vi "Curtin1_ReadWriteFRFGraphData.vi"(8 "Type":T3 items=["FRF", "rad phase unwrapped", "deg phase unwrapped", "rad phase wrapped", "deg phase wrapped", "White Plots", "MJ Map", "Real and Imaginary"], 9 "FRF":refnum<vi>, 11 "Task":enum16{"Read", "Save"}(ring)) -> (0 "y log?":bool, 1 "x log?":bool, 2 "dB":dbl)   [LabVIEW 2022 SP3]
uses:
  GraphType.ctl
  <vilib>/Utility/miscctls.llb/LVRangeTypeDef.ctl
  Mic/Mic_Global.vi
panel:
  out "Graph settings":T2
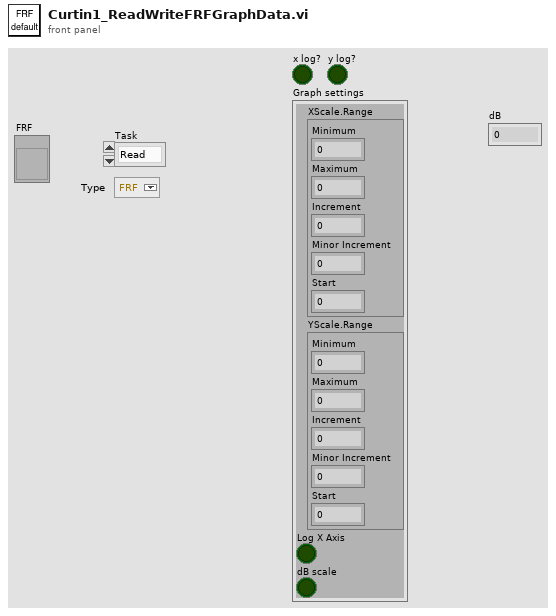
[diagram p1: front panel]
types:
  T1 = typedef "LVRangeTypeDef.ctl" = cluster{"Minimum":dbl, "Maximum":dbl, "Increment":dbl, "Minor Increment":dbl, "Start":dbl}
  T2 = cluster{"XScale.Range":T1, "YScale.Range":T1, "Log X Axis":bool, "dB scale":bool}
  T3 = typedef "GraphType.ctl" = u16
  T4 = cluster{"Alerts":bool, "Log X Axis":bool, "dB scale":bool, "Averaging":bool, "Fade":dbl, "Centroids?":bool}
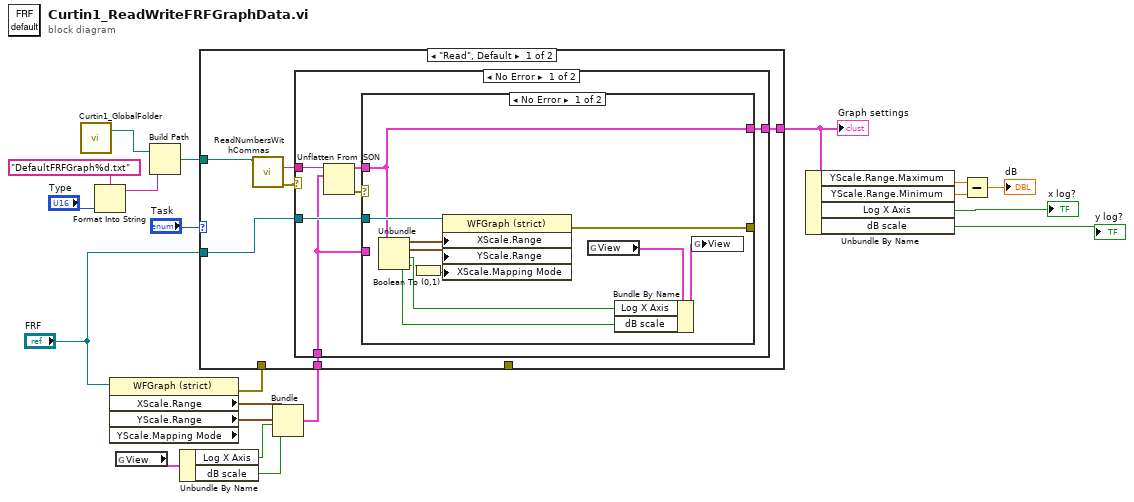
[diagram p0: block diagram]
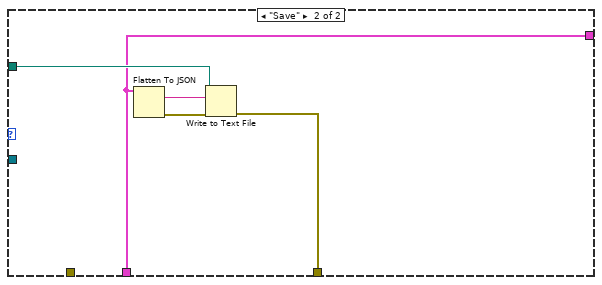
[diagram p4: hidden frame]
diagram:
  n1 = call "Curtin1_GlobalFolder.vi"() -> ("LabVIEW Data Path"=w20:path)  [unwired: 1 in, 1 out]
  n2 = Format Into String(format string="DefaultFRFGraph%d.txt" ("name or relative path"), "Type") -> (resulting string=w6:string)  [unwired: 2 in, 1 out]
  n3 = property class="WFGraph (strict)" props=["XScale", "Range", "YScale", "Range", "YScale", "Mapping Mode"](reference="FRF") -> (error out=w13:errorcluster, "XScale.Range"=w17:T1, "YScale.Range"=w16:T1)  [unwired: 1 in, 2 out]
  n4 = global read "Mic_Global.vi" "View"() -> (w5:T4)
  n5 = Build Path(base path=w20, name or relative path=w6) -> (appended path=w19:path)
  n6 = Unbundle By Name(w5) -> ("Log X Axis"=w4:bool, "dB scale"=w3:bool)
  n7 = Bundle("XScale.Range"=w17, "YScale.Range"=w16, "Log X Axis"=w4, "dB scale"=w3) -> (w15:T2)  [unwired: 1 in]
  n8 = case shown="\"Read\", Default" "Task" {
    tunnel: w19 -> [w23 w47]
    tunnel: [_ w46] -> _
    tunnel: w15 -> [w26 w45]
    tunnel: "FRF" -> [w25 _]
    tunnel: w13 -> [_ _]
    tunnel: [w24 w45] -> w12
    frame "Read", Default {
      n9 = call "ReadNumbersWithCommas.vi"("file (use dialog)"=w23) -> ("error out"=w22:errorcluster, "text"=w21:string)  [unwired: 7 in, 2 out]
      n10 = case shown="No Error" w22 {
        tunnel: w21 -> [w32 _]
        tunnel: w26 -> [w27 w44]
        tunnel: w25 -> [w29 _]
        tunnel: [w28 w44] -> w24
        frame No Error {
          n11 = Unflatten From JSON(JSON string=w32, type and defaults=w27) -> (value=w30:T2, error out=w31:errorcluster)  [unwired: 5 in]
          n12 = case shown="No Error" w31 {
            tunnel: w30 -> [w38 _]
            tunnel: w29 -> [w42 _]
            tunnel: [w39 _] -> _
            tunnel: [w38 w43] -> w28
            tunnel: w27 -> [_ w43]
            frame No Error {
              n13 = Unbundle(w38) -> ("XScale.Range"=w41:T1, "YScale.Range"=w40:T1, "Log X Axis"=w35:bool, "dB scale"=w34:bool)
              n14 = Boolean To (0,1)(Boolean=w34) -> (0, 1=w33:i16)
              n15 = property class="WFGraph (strict)"(reference=w42, "XScale.Range"=w41, "YScale.Range"=w40, "XScale.Mapping Mode"=w33) -> (error out=w39:errorcluster)  [unwired: 1 in, 1 out]
              n16 = global read "Mic_Global.vi" "View"() -> (w37:T4)
              n17 = Bundle By Name(cluster=w37, "Log X Axis"=w35, "dB scale"=w34) -> (w36:T4)
              n18 = global write "Mic_Global.vi" "View"(w36) -> ()
            }
            frame Error {
            }
          }
        }
        frame Error {
        }
      }
    }
    frame "Save" {
      n19 = Flatten To JSON(anything=w45) -> (JSON string=w49:string, 11:w48:errorcluster)  [unwired: 2 in]
      n20 = Write to Text File(file (use dialog)=w47, text=w49, error in=w48) -> (error out=w46:errorcluster)  [unwired: 1 in, 2 out]
    }
  }
  "Graph settings" <- w12
  n21 = Unbundle By Name(w12) -> ("YScale.Range.Maximum"=w10:dbl, "YScale.Range.Minimum"=w11:dbl, "Log X Axis"=→"x log?":bool, "dB scale"=→"y log?":bool)
  n22 = Subtract(x=w10, y=w11) -> (x-y=→"dB":dbl)
